vi "GlobalMesaurementOut.vi"() -> ()   [LabVIEW 2013]
panel:
  in  "PathData":string
  in  "Meta":dbl[](array[numeric])
  in  "Data":i32[](array[numeric])
  in  "Intensity":dbl[](array[numeric])
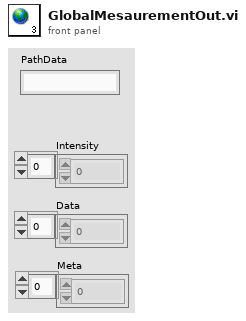
[diagram p1: front panel]
diagram:
